vi "Profile.vi"(11 "Queue In":refnum<queue>) -> ()   [LabVIEW 2013, in "main.lvlib"]
uses:
  main.lvlib
  Controls/Reference AE Control.ctl
  Controls/Enum Save Action Events.ctl
  Controls/Enum Variables.ctl
panel:
  in  "Search Patient ID":string caption="Søg"
  in  "Listbox Patient ID":i32(listbox)=-1 caption="CPR Number"
  in  "Query Worklist":bool
  in  "Add Patient ID Btn":bool caption="Add CPR"
  in  "ListboxOperator":i32(listbox)=-1 caption="Operator"
  in  "ListboxDoctor":i32(listbox)=-1 caption="Doctor"
  in  "StopProfile":bool
  out "HospitalDepartment":string caption="Afdeling"
  in  "CommentStr":string caption="Kommentar"
  out "HospitalAddress":string caption="Adresse"
  in  "EditHospInfo":bool
  out "HospitalName":string caption="Hospital"
  in  "Name":string caption="Navn"
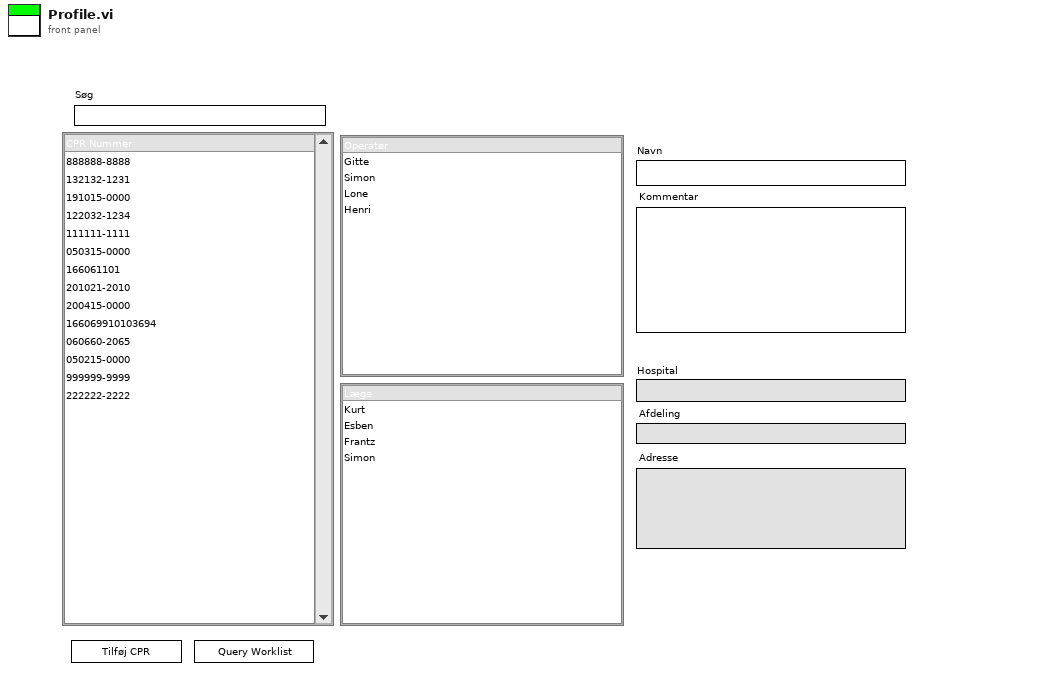
[diagram p1: front panel]
types:
  T1 = typedef "main.lvlib/Reference AE Control.ctl" = enum16{"Initialize", "Set Menu", "Set Profile", "Set Configuration", "Set Configuration_old", "Set Configuration_new", "Set Configuration Method", "Set Acquisition", "Set Data", "Set Journal", "Get"}
  T2 = typedef "main.lvlib/Enum Variables.ctl" = enum16{"SetAcqFilter", "GetAcqFilter", "Set Filter", "Get Filter", "Set Height", "Get Height", "Set Recorded Height", "Get Recorded Height", "Set Blue Pressure", "Get Blue Pressure", "Set Red Pressure", "Get Red Pressure", "Init", "Reset Pressure", "Set Red Cursors", "Get Red Cursors", "Set Blue Cursors", "Get Blue Cursors", "Set Language", "Get Language", "Set Active Graphs", "Get ActiveGraphs", "Set Method", "Get Method", "Set Encryption", "Get Encryption", "Set ExcelVersion", "Get ExcelVersion", "Set DICOM Avail", "Get DICOM Avail", "Set DICOM Encode", "Get DICOM Encode", "Set JournalExport", "Get JournalExport", "Set Sequence", "Get Sequence", "Set DAQ Connected", "Get DAQ Connected", "Set Current Graph", "Get Current Graph", "Set General Settings", "Get Hyphenation", "Set Arm Calc Method", "Get Arm Calc Method", "Set Dicom Tags", "Get Dicom Tags", "Set BT Serial", "Get BT Serial", "Set BT Accepted Serials", "Get BT Accepted Serials", "Get BT License", "Set BT License"}
  T3 = typedef "main.lvlib/Enum Save Action Events.ctl" = enum16{"LoadReportPath", "SaveReportPath", "Load Graph Path", "Save Graph Path", "LoadDataPath", "SaveDataPath", "Load Template Path", "Save Template Path", "Load PressureFactor", "Save PressureFactor", "Init", "Load Listbox", "Save Listbox", "LoadHospInfo", "SaveHospInfo", "Load DICOM Activation", "Save DICOM Activation", "LoadDICOMInfoWL", "SaveDICOMInfoWL", "LoadDICOMInfoPACS", "SaveDICOMInfoPACS", "Load ArmCalcMethod", "Save ArmCalcMethod", "LoadItemTags", "SaveItemTags", "LoadDICOMEncoding", "SaveDICOMEncoding", "LoadJournalType", "SaveJournalType", "LoadAcqFilterType", "SaveAcqFilterType", "Load Sequence", "Save Sequence", "Load Acquisition Mode", "Save Acquisition Mode", "Load General Settings", "Save General Settings", "Load Language", "Save Language", "Load Dicom Tags", "Save Dicom Tags", "Load BT Serial", "Save BT Serial", "Load BT License", "Save BT License"}
  T4 = cluster{"Name":string, "Address":string, "Department":string}
  T5 = cluster{"Search Patient ID":refnum<vi>, "Name":refnum<vi>, "CommentStr":refnum<vi>, "Listbox Patient ID":refnum<vi>, "ListboxDoctor":refnum<vi>, "ListboxOperator":refnum<vi>, "HospitalName":refnum<vi>, "HospitalDepartment":refnum<vi>, "HospitalAddress":refnum<vi>, "EditHospInfo":refnum<vi>, "Add Patient ID Btn":refnum<vi>, "Query Worklist":refnum<vi>}
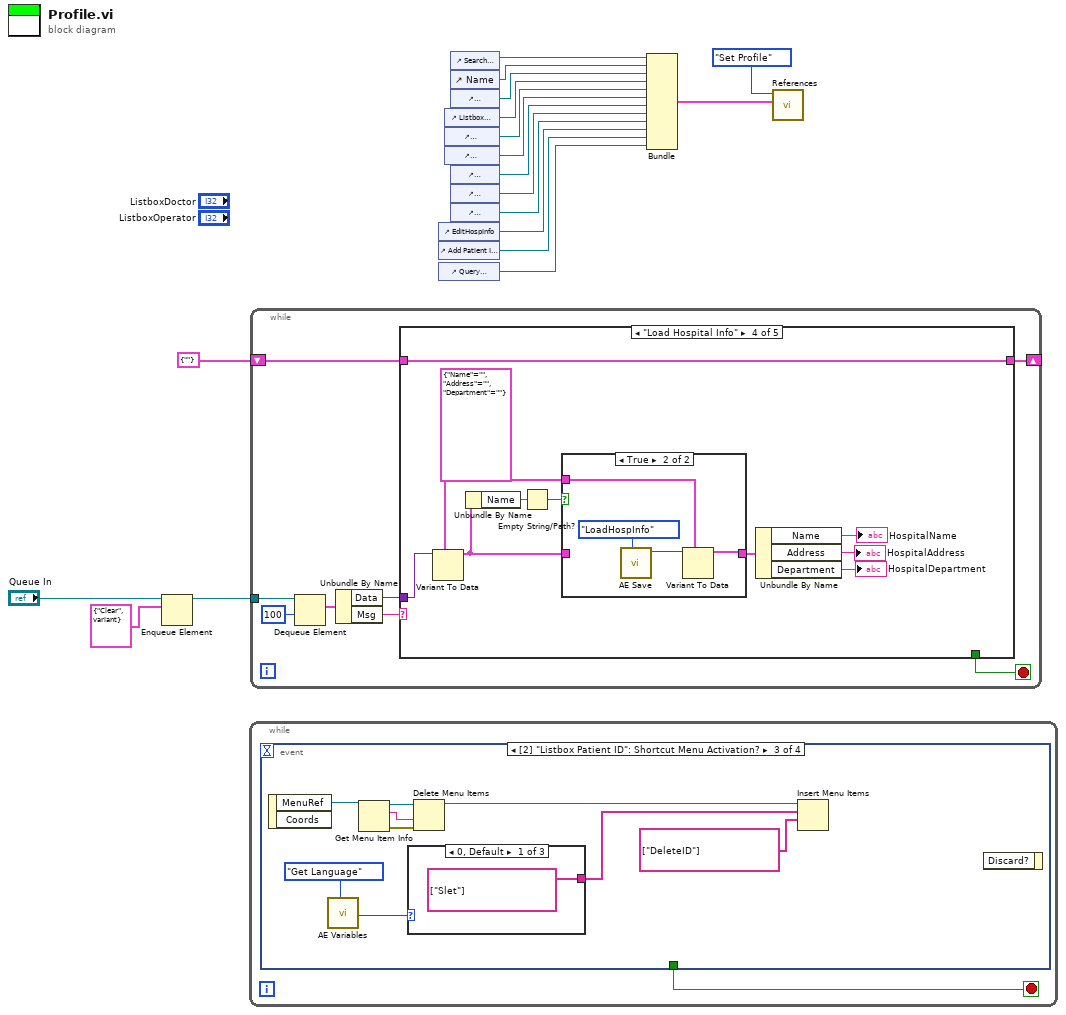
[diagram p0: block diagram]
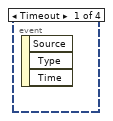
[diagram p2: hidden frame]
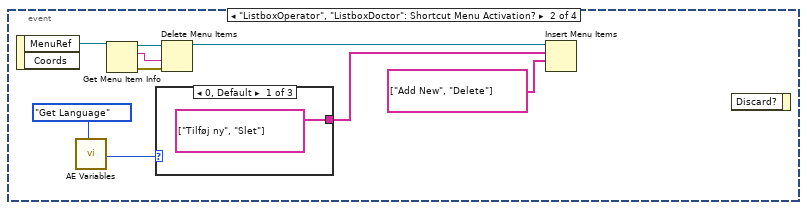
[diagram p3: hidden frame]
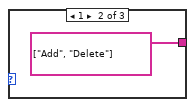
[diagram p4: hidden frame]
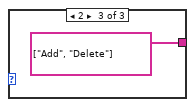
[diagram p5: hidden frame]
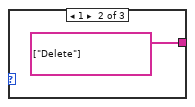
[diagram p6: hidden frame]
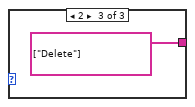
[diagram p7: hidden frame]
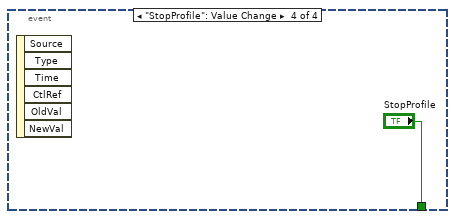
[diagram p8: hidden frame]
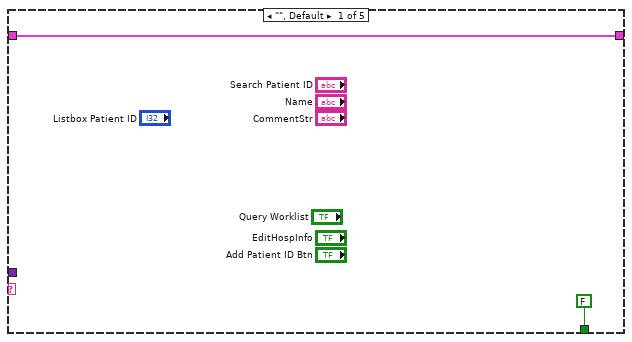
[diagram p9: hidden frame]
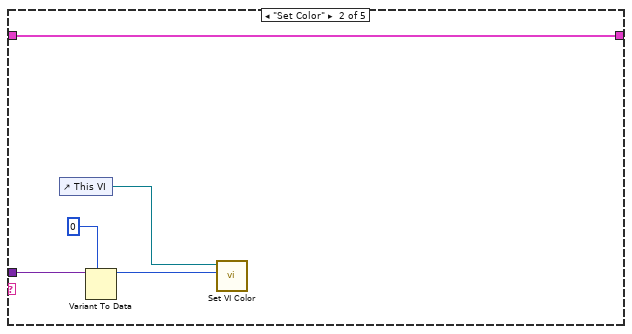
[diagram p10: hidden frame]
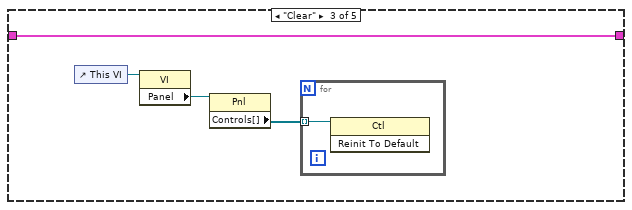
[diagram p11: hidden frame]
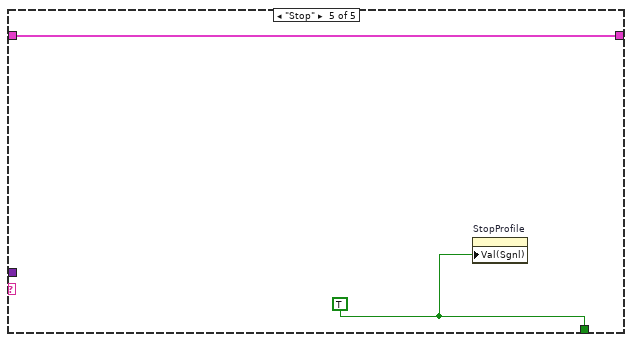
[diagram p13: hidden frame]
diagram:
  n1 = Enqueue Element(queue="Queue In", element=cluster{"Msg":string, "Data":variant} {"Msg"="Clear", "Data"=variant}) -> (queue out=w2:refnum<queue>)  [unwired: 2 in, 2 out]
  n2 = while {
    stop <- w19 stop-if-true
    n3 = event shown="[2] \"Listbox Patient ID\": Shortcut Menu Activation?" {
      selector: _ -> [_ _ _ _]
      dyn-events: _ -> [_ _ _ _]
      timeout: _ -> [_ _ _ _]
      tunnel: [_ _ _ "StopProfile"] -> w19
      event Timeout {
        n4 = event-data() -> ()  [unwired: 1 in, 3 out]
      }
      event "ListboxOperator", "ListboxDoctor": Shortcut Menu Activation? {
        n5 = event-data() -> ("MenuRef"=w28:refnum<k9>)  [unwired: 1 in, 1 out]
        n6 = call "AE Variables.vi"("Action"=Enum_Variables."Get Language") -> ("RingOut"=w20:u16)  [unwired: 11 in, 7 out]
        n7 = Get Menu Item Info(11:w28) -> (0:w25:errorcluster, 2:w26:string, 3:w27:refnum<k9>)  [unwired: 2 in, 4 out]
        n8 = case shown="0, Default" w20 {
          tunnel: [string[] ["Tilføj ny", "Slet"] string[] ["Add", "Delete"] string[] ["Add", "Delete"]] -> w23
          frame 0, Default {
          }
          frame 1 {
          }
          frame 2 {
          }
        }
        n9 = Delete Menu Items(6:w25, 7:w26, 9:w27) -> (3:w24:refnum<k9>)  [unwired: 1 in, 1 out]
        n10 = Insert Menu Items(7:string[] ["Add New", "Delete"], 8:w23, 9:w24) -> ()  [unwired: 3 in, 3 out]
        n11 = event-data() -> ()  [unwired: 2 in, 1 out]
      }
      event "Listbox Patient ID": Shortcut Menu Activation? {
        n12 = event-data() -> ("MenuRef"=w40:refnum<k9>)  [unwired: 1 in, 1 out]
        n13 = call "AE Variables.vi"("Action"=Enum_Variables."Get Language") -> ("RingOut"=w32:u16)  [unwired: 11 in, 7 out]
        n14 = Get Menu Item Info(11:w40) -> (0:w37:errorcluster, 2:w38:string, 3:w39:refnum<k9>)  [unwired: 2 in, 4 out]
        n15 = case shown="0, Default" w32 {
          tunnel: [string[] ["Slet"] string[] ["Delete"] string[] ["Delete"]] -> w35
          frame 0, Default {
          }
          frame 1 {
          }
          frame 2 {
          }
        }
        n16 = Delete Menu Items(6:w37, 7:w38, 9:w39) -> (3:w36:refnum<k9>)  [unwired: 1 in, 1 out]
        n17 = Insert Menu Items(7:string[] ["DeleteID"], 8:w35, 9:w36) -> ()  [unwired: 3 in, 3 out]
        n18 = event-data() -> ()  [unwired: 2 in, 1 out]
      }
      event "StopProfile": Value Change {
        n19 = event-data() -> ()  [unwired: 1 in, 6 out]
      }
    }
  }
  n20 = while {
    tunnel: w2 -> [w51]
    shift-right: [w48] -> _
    shift-left: cluster{string} {""} -> [w49]
    stop <- w52 stop-if-true
    n21 = Dequeue Element(queue=w51, timeout in ms (-1)=100) -> (element=w50:cluster{"Msg":string, "Data":variant})  [unwired: 1 in, 3 out]
    n22 = Unbundle By Name(w50) -> ("Data"=w47:variant, "Msg"=w45:string)
    n23 = case shown="\"Load Hospital Info\"" w45 {
      tunnel: [FALSE _ _ _ w80] -> w52
      tunnel: w49 -> [w53 w55 w60 w74 w81]
      tunnel: [w53 w55 w60 w74 w81] -> w48
      tunnel: w47 -> [_ w58 _ w72 _]
      frame "", Default {
      }
      frame "Set Color" {
        n24 = control-ref of="This VI"() -> (w59:refnum<vi>)
        n25 = Variant To Data(type=u32 0 ("Pane Color"), Variant=w58) -> (data=w56:u32)  [unwired: 1 in, 1 out]
        n26 = call "Set VI Color.vi"("Pane Color"=w56, "VI in"=w59) -> ()  [unwired: 10 in]
      }
      frame "Clear" {
        n27 = control-ref of="This VI"() -> (w63:refnum<vi>)
        n28 = property class="VI"(reference=w63) -> ("Panel"=w62:refnum<vi>)  [unwired: 1 in, 2 out]
        n29 = property class="Pnl"(reference=w62) -> ("Controls[]"=w61:refnum<vi>[])  [unwired: 1 in, 2 out]
        n30 = for {
          tunnel: w61 -> [w64] mode=indexing
          n31 = invoke class="Ctl" method="Reinit To Default"(reference=w64) -> ()  [unwired: 2 in, 3 out]
        }
      }
      frame "Load Hospital Info" {
        w65 = T4 {"Name"="", "Address"="", "Department"=""} ("output cluster")
        n32 = Variant To Data(type=w65, Variant=w72) -> (data=w67:T4)  [unwired: 1 in, 1 out]
        n33 = Unbundle By Name(w67) -> ("Name"=w69:string)
        n34 = Empty String/Path?(string/path=w69) -> (empty?=w68:bool)
        n35 = case shown="True" w68 {
          tunnel: w67 -> [w75 _]
          tunnel: [w75 w78] -> w66
          tunnel: w65 -> [_ w76]
          frame False {
          }
          frame True {
            n36 = call "AE Save.vi"("Action"=Enum_Save_Action_Events."LoadHospInfo") -> ("Anything"=w77:variant)  [unwired: 8 in, 1 out]
            n37 = Variant To Data(type=w76, Variant=w77) -> (data=w78:T4)  [unwired: 1 in, 1 out]
          }
        }
        n38 = Unbundle By Name(w66) -> ("Name"=→"HospitalName":string, "Address"=→"HospitalAddress":string, "Department"=→"HospitalDepartment":string)
      }
      frame "Stop" {
        w80 = TRUE
        n39 = property on="StopProfile" class="Bool (strict)"("Val(Sgnl)"=w80) -> ()  [unwired: 2 in, 2 out]
      }
    }
  }
  n40 = control-ref of="EditHospInfo"() -> (w9:refnum<vi>)
  n41 = control-ref of="Add Patient ID Btn"() -> (w8:refnum<vi>)
  n42 = control-ref of="Query Worklist"() -> (w1:refnum<vi>)
  n43 = control-ref of="Listbox Patient ID"() -> (w15:refnum<vi>)
  n44 = control-ref of="ListboxDoctor"() -> (w14:refnum<vi>)
  n45 = control-ref of="ListboxOperator"() -> (w13:refnum<vi>)
  n46 = control-ref of="Search Patient ID"() -> (w18:refnum<vi>)
  n47 = control-ref of="Name"() -> (w17:refnum<vi>)
  n48 = control-ref of="CommentStr"() -> (w16:refnum<vi>)
  n49 = control-ref of="HospitalName"() -> (w12:refnum<vi>)
  n50 = control-ref of="HospitalDepartment"() -> (w11:refnum<vi>)
  n51 = control-ref of="HospitalAddress"() -> (w10:refnum<vi>)
  n52 = Bundle("Search Patient ID"=w18, "Name"=w17, "CommentStr"=w16, "Listbox Patient ID"=w15, "ListboxDoctor"=w14, "ListboxOperator"=w13, "HospitalName"=w12, "HospitalDepartment"=w11, "HospitalAddress"=w10, "EditHospInfo"=w9, "Add Patient ID Btn"=w8, "Query Worklist"=w1) -> (w6:T5)  [unwired: 1 in]
  n53 = call "References.vi"("variant"=w6, "Reference AE Control"=Reference_AE_Control."Set Profile") -> ()  [unwired: 8 in, 2 out]
